vi "GcodeXY_Rotation.vi"(4 "error in":errorcluster, 6 "AngleInDeg":dbl, 7 "GCodeIn":string="G1X-10.813Y18.752F100") -> (0 "error out 2":errorcluster, 3 "GCodeOut":string)   [LabVIEW 2019]
uses:
  <vilib>/Analysis/coordinate.llb/2D Cartesian Coordinate Rotation (Scalar).vi
  <vilib>/Analysis/NI_AALPro.lvlib
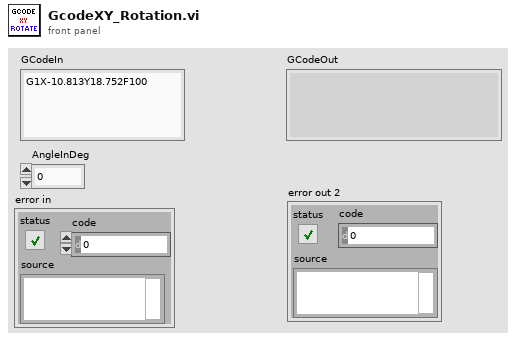
[diagram p1: front panel]
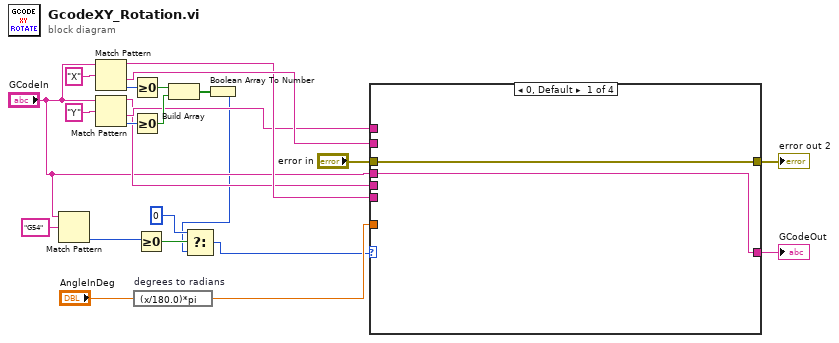
[diagram p0: block diagram]
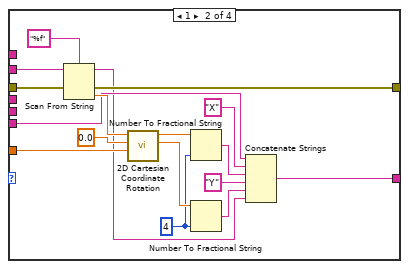
[diagram p2: hidden frame]
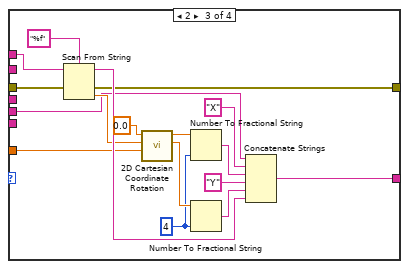
[diagram p3: hidden frame]
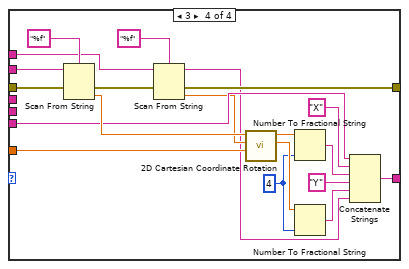
[diagram p4: hidden frame]
diagram:
  n1 = Match Pattern(string="GCodeIn", regular expression="G54") -> (offset past match=w5:i32)  [unwired: 1 in, 3 out]
  n2 = Match Pattern(string="GCodeIn", regular expression="X") -> (before substring=w10:string, after substring=w14:string, offset past match=w21:i32)  [unwired: 1 in, 1 out]
  n3 = Match Pattern(string="GCodeIn", regular expression="Y") -> (before substring=w8:string, after substring=w9:string, offset past match=w19:i32)  [unwired: 1 in, 1 out]
  n4 = Greater Or Equal To 0?(x=w21) -> (x >= 0?=w18:bool)
  n5 = Greater Or Equal To 0?(x=w19) -> (x >= 0?=w17:bool)
  n6 = expression code="(x/180.0)*pi" "degrees to radians"("AngleInDeg") -> (w13:dbl)
  n7 = Greater Or Equal To 0?(x=w5) -> (x >= 0?=w4:bool)
  n8 = Build Array(w18, w17) -> (w16:bool[])
  n9 = Boolean Array To Number(Boolean array=w16) -> (number=w1:u8)
  n10 = Select(t=u8 0 ("f"), s=w4, f=w1) -> (s? t:f=w3:u8)
  n11 = case shown="0, Default" w3 {
    tunnel: "GCodeIn" -> [w25 _ _ _]
    tunnel: [w25 w29 w43 w61] -> w15
    tunnel: w14 -> [_ w41 _ w69]
    tunnel: w13 -> [_ w37 w48 w67]
    tunnel: "error in" -> [w24 w34 w49 w68]
    tunnel: [w24 w33 w47 w64] -> w11
    tunnel: w10 -> [_ w32 _ w70]
    tunnel: w9 -> [_ _ w50 w60]
    tunnel: w8 -> [_ _ w44 _]
    frame 0, Default {
    }
    frame 1 {
      w38 = i16 4 ("precision (6)")
      n12 = Scan From String(format string="%f", input string=w41, error in=w34) -> (remaining string=w26:string, error out=w33:errorcluster, output 1=w36:dbl)  [unwired: 2 in, 1 out]
      n13 = call-poly <vilib>:"2D Cartesian Coordinate Rotation.vi"("theta"=w37, "y"=0.0, "x"=w36) -> ("y out"=w40:dbl, "x out"=w39:dbl)  [unwired: 6 in, 1 out]
      n14 = Number To Fractional String(number=w39, precision (6)=w38) -> (F-format string=w30:string)  [unwired: 2 in]
      n15 = Number To Fractional String(number=w40, precision (6)=w38) -> (F-format string=w27:string)  [unwired: 2 in]
      n16 = Concatenate Strings(w32, "X" ("regular expression"), w30, "Y" ("regular expression"), w27, w26) -> (w29:string)
    }
    frame 2 {
      w56 = i16 4 ("precision (6)")
      n17 = Scan From String(format string="%f", input string=w50, error in=w49) -> (remaining string=w51:string, error out=w47:errorcluster, output 1=w46:dbl)  [unwired: 2 in, 1 out]
      n18 = call-poly <vilib>:"2D Cartesian Coordinate Rotation.vi"("theta"=w48, "y"=w46, "x"=0.0 ("y")) -> ("y out"=w58:dbl, "x out"=w57:dbl)  [unwired: 6 in, 1 out]
      n19 = Number To Fractional String(number=w57, precision (6)=w56) -> (F-format string=w54:string)  [unwired: 2 in]
      n20 = Number To Fractional String(number=w58, precision (6)=w56) -> (F-format string=w52:string)  [unwired: 2 in]
      n21 = Concatenate Strings(w44, "X" ("regular expression"), w54, "Y" ("regular expression"), w52, w51) -> (w43:string)
    }
    frame 3 {
      w76 = i16 4 ("precision (6)")
      n22 = Scan From String(format string="%f", input string=w69, error in=w68) -> (error out=w65:errorcluster, output 1=w75:dbl)  [unwired: 2 in, 2 out]
      n23 = Scan From String(format string="%f", input string=w60, error in=w65) -> (remaining string=w62:string, error out=w64:errorcluster, output 1=w63:dbl)  [unwired: 2 in, 1 out]
      n24 = call-poly <vilib>:"2D Cartesian Coordinate Rotation.vi"("theta"=w67, "y"=w63, "x"=w75) -> ("y out"=w78:dbl, "x out"=w77:dbl)  [unwired: 6 in, 1 out]
      n25 = Number To Fractional String(number=w77, precision (6)=w76) -> (F-format string=w73:string)  [unwired: 2 in]
      n26 = Number To Fractional String(number=w78, precision (6)=w76) -> (F-format string=w71:string)  [unwired: 2 in]
      n27 = Concatenate Strings(w70, "X" ("regular expression"), w73, "Y" ("regular expression"), w71, w62) -> (w61:string)
    }
  }
  "GCodeOut" <- w15
  "error out 2" <- w11
